vi "VisualizeNHRDC0.vi"() -> ()   [LabVIEW 2018, in "Visualization.lvlib" / "VisualizeAcPwr.lvclass"]
uses:
  VisualizeAcPwr.lvclass
  <vilib>/event_ctls.llb/usereventprio.ctl
  VisualizeBase/VisualizeBase_class/Requests/clUserEventType.ctl
  <vilib>/Utility/error.llb/Error Cluster From Error Code.vi
  <vilib>/ErrorRing/Error Ring.xnode
  VisualizeBase/VisualizeBase_class/VisualizeBase.lvclass
  <userlib>/NIST/NISTErrorLib/NISTErrorLib.lvlib
  AcPwr/AcPwrModule/AcPwrModule.lvlib
panel:
  out "Incorrect DataType?":bool
  in  "PluginName":string="AcPwr.NHRDC0"
  in  "PlotYAxis":u32[](array[numeric])=[0, 1, 0] max=1
  out "NHRDC":waveform(dbl)[](graph)
  out "ErrorArray":errorcluster[](array[cluster])
  in  "QueuName":string="NHRDCVQ"
  in  "btnStop":bool
  in  "btnReset":bool
  in  "btnClear":bool
  # "0=Left Axis and 1=Right Axis"
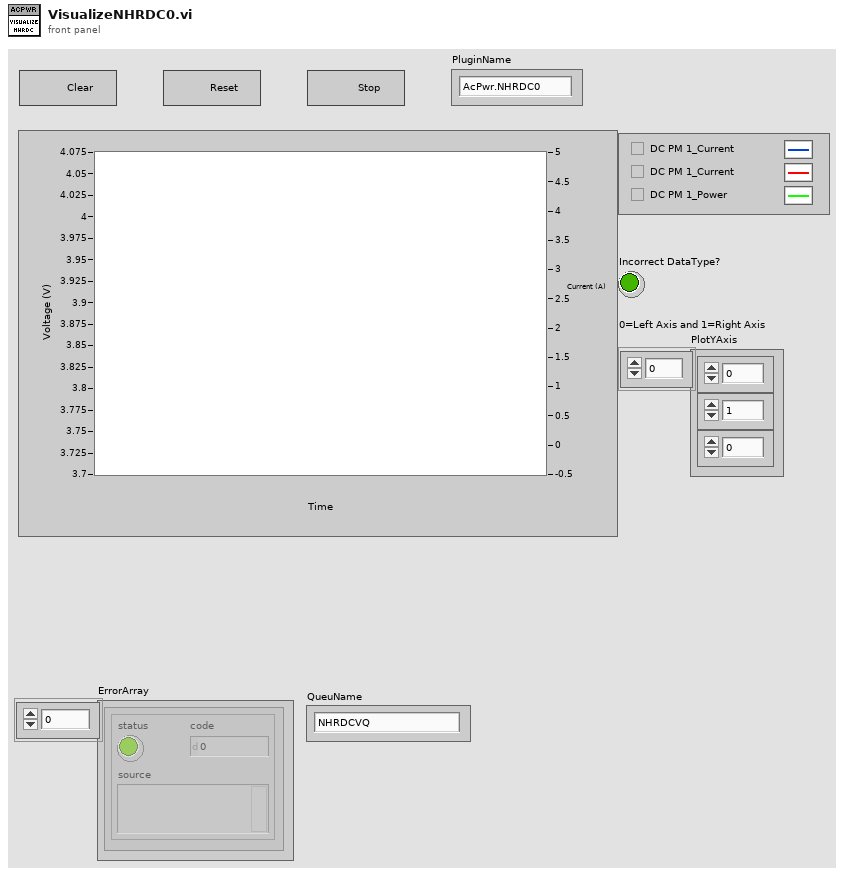
[diagram p1: front panel]
types:
  T1 = typedef "Visualization.lvlib/VisualizeBase.lvclass/clRequestEvents.ctl" = cluster{"StopRequest":refnum<user-event>, "ResetRequest":refnum<user-event>}
  T2 = typedef "AcPwrModule.lvlib/clBroadcastEvents.ctl" = cluster{"DidInit":refnum<user-event>, "StatusUpdate":refnum<user-event>, "ErrorReport":refnum<user-event>, "DidStop":refnum<user-event>, "PathToINI":refnum<user-event>, "Measurements":refnum<user-event>, "LoadConfigFile":refnum<user-event>, "GetSettings":refnum<user-event>, "SetSettings":refnum<user-event>, "GetType&ID":refnum<user-event>, "GotSettings":refnum<user-event>}
  T3 = typedef "Visualization.lvlib/VisualizeBase.lvclass/clUserEventType.ctl" = cluster{"BusIndex":i8, "Data":variant}
  T4 = typedef "usereventprio.ctl" = enum32{"high priority", "normal priority"}
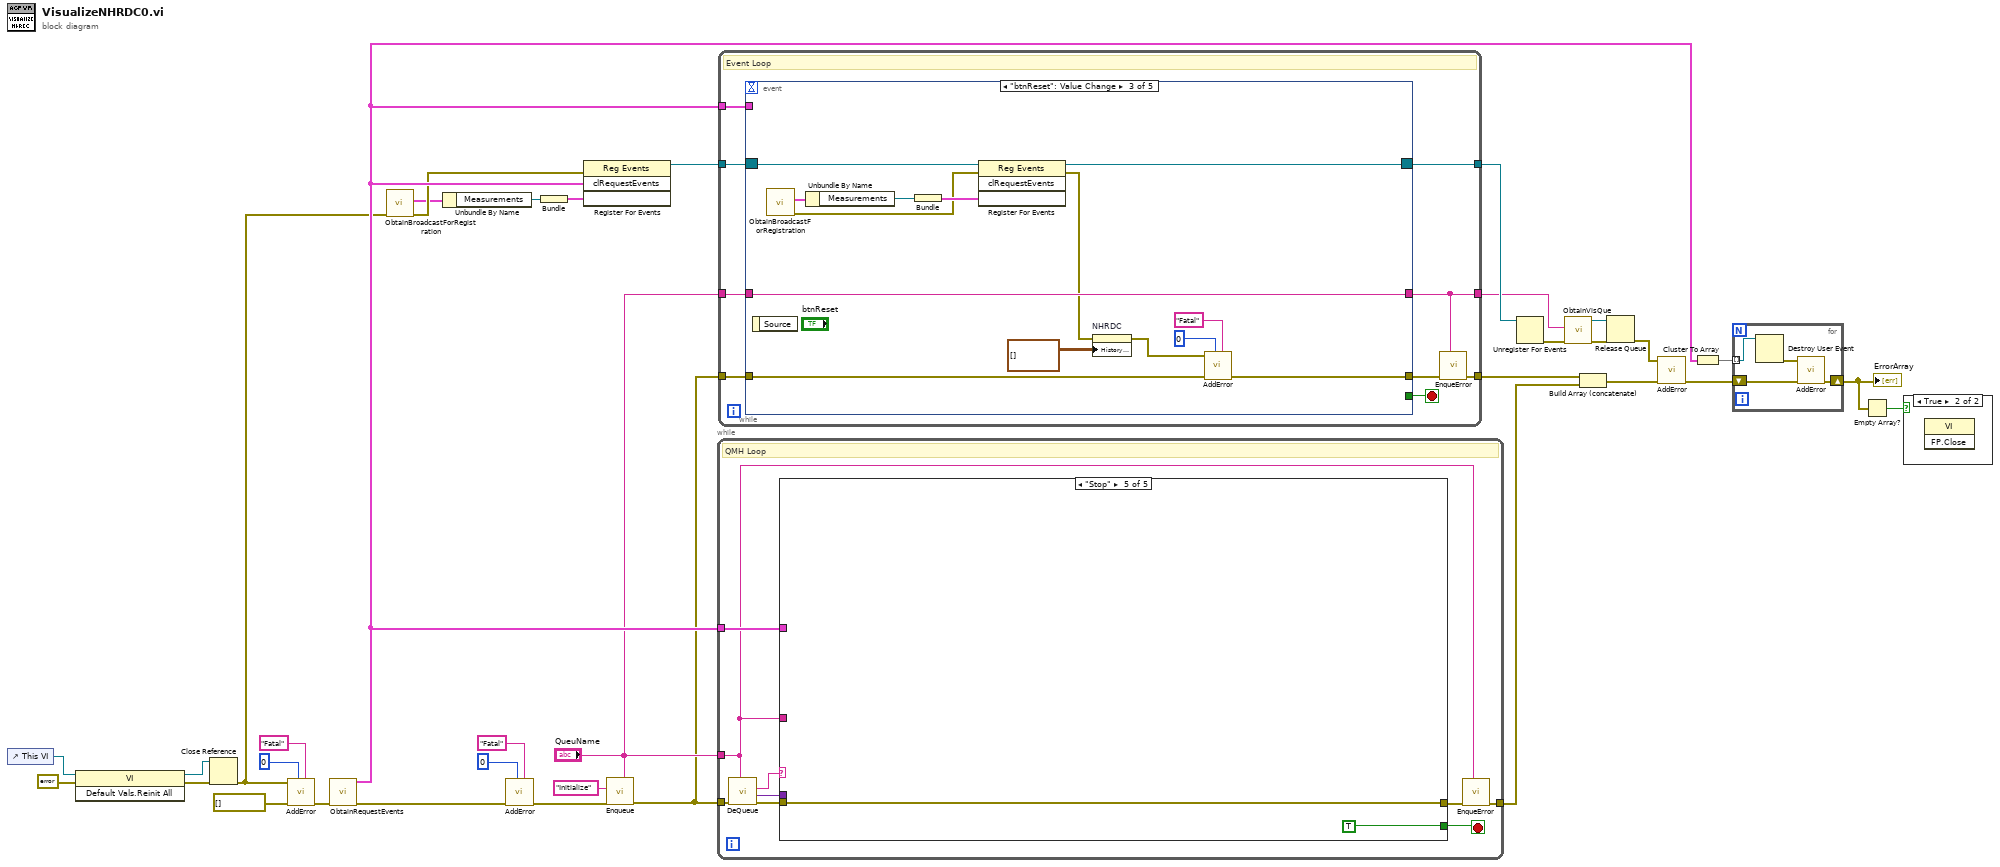
[diagram p0: block diagram]
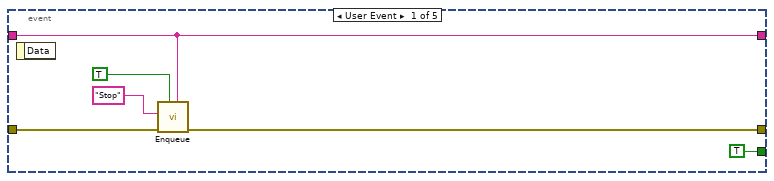
[diagram p2: hidden frame]
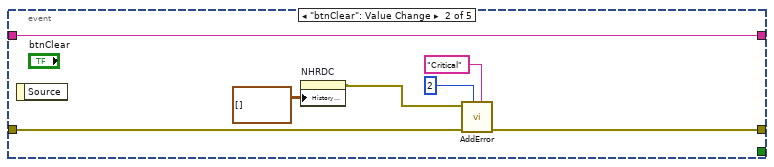
[diagram p3: hidden frame]
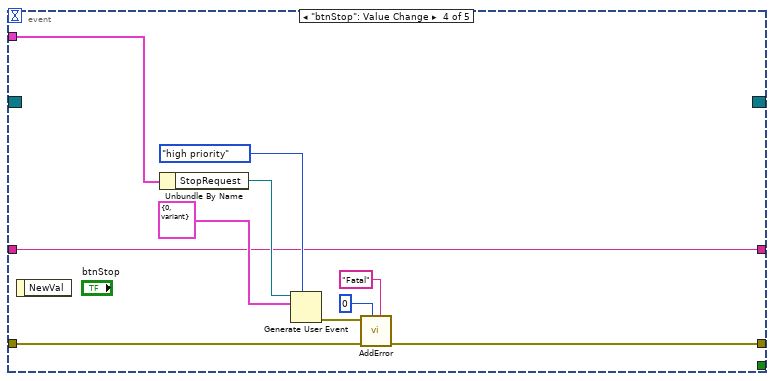
[diagram p4: hidden frame]
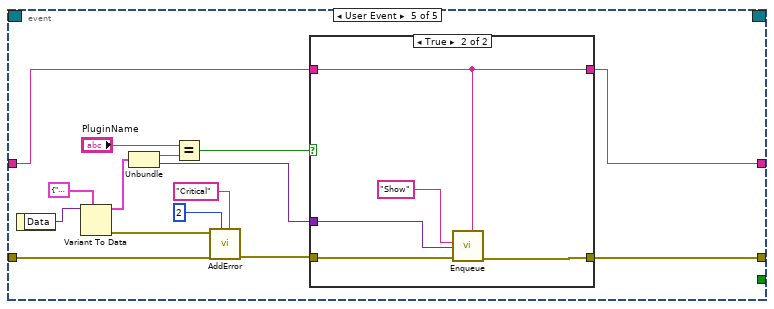
[diagram p5: hidden frame]
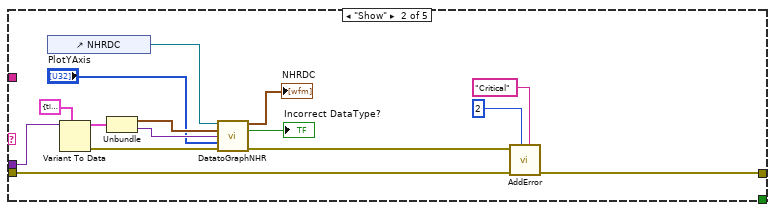
[diagram p8: hidden frame]
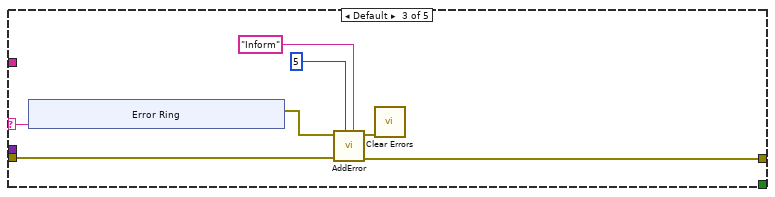
[diagram p9: hidden frame]
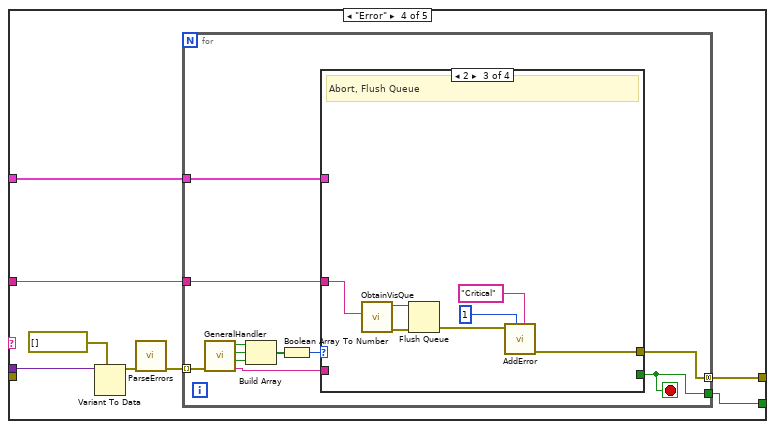
[diagram p10: hidden frame]
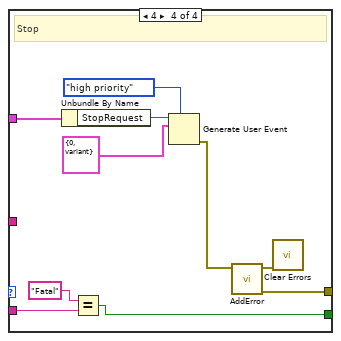
[diagram p13: hidden frame]
diagram:
  n1 = control-ref of="This VI"() -> (w18:refnum<vi>)
  n2 = invoke class="VI" method="Default Vals.Reinit All"(reference=w18, error in=errorcluster {"status"=FALSE, "code"=0, "source"=""} ("error in (no error)")) -> (reference out=w15:refnum<vi>, error out=w16:errorcluster)  [unwired: 1 in, 1 out]
  n3 = Close Reference(reference=w15, error in (no error)=w16) -> (error out=w13:errorcluster)
  n4 = call <userlib>:"AddError.vi"("Severity"="Fatal" ("String"), "Priority"=u8 0, "ErrorArray"=errorcluster[] [], "error in (no error)"=w13) -> ("ErrorArray"=w33:errorcluster[])  [unwired: 6 in, 1 out]
  n5 = call "ObtainRequestEvents.vi"("Error"=w33) -> ("Error"=w3:errorcluster[], "clRequestEvents"=w22:T1)  [unwired: 9 in]
  n6 = call "ObtainBroadcastForRegistration.vi"("error in (no error)"=w13) -> ("error out"=w12:errorcluster, "clBroadcastEvents"=w11:T2)  [unwired: 9 in]
  n7 = Unbundle By Name(w11) -> ("Measurements"=w20:refnum<user-event>)
  n8 = call <userlib>:"AddError.vi"("Severity"="Fatal" ("String"), "Priority"=u8 0, "ErrorArray"=w3) -> ("ErrorArray"=w2:errorcluster[])  [unwired: 7 in, 1 out]
  n9 = Bundle("Measurements"=w20) -> (w19:cluster{"Measurements":refnum<user-event>})  [unwired: 1 in]
  n10 = register-events(error in=w12, w22, w19) -> (reference out=w34:refnum<event-registration>)  [unwired: 1 in, 1 out]
  n11 = call "Enqueue.vi"("QueName"="QueuName", "Error"=w2, "Message"="Initialize") -> ("Error"=w1:errorcluster[])  [unwired: 8 in]
  n12 = while {
    tunnel: w1 -> [w44]
    tunnel: [w38] -> w29
    tunnel: "QueuName" -> [w36]
    tunnel: w22 -> [w37]
    stop <- w39 stop-if-true
    # "QMH Loop"
    n13 = call "DeQueue.vi"("QueName"=w36, "Error"=w44) -> ("Error"=w41:errorcluster[], "Data"=w42:variant, "Message"=w43:string)  [unwired: 7 in]
    n14 = case shown="\"Stop\"" w43 {
      selector: w43 -> [_ _ w67 _ _]
      tunnel: w42 -> [_ w53 _ w82 _]
      tunnel: w41 -> [w45 w56 w65 _ w111]
      tunnel: [w45 w60 w64 w78 w111] -> w40
      tunnel: [_ _ _ w77 TRUE] -> w39
      tunnel: w37 -> [_ _ _ w76 _]
      tunnel: w36 -> [_ _ _ w75 _]
      frame "Initialize" {
      }
      frame "Show" {
        n15 = control-ref of="NHRDC"() -> (w52:refnum<vi>)
        n16 = Variant To Data(type=cluster{timestamp, "Data":variant} {timestamp(0 s since 1904-01-01), "Data"=variant}, Variant=w53) -> (data=w55:cluster{timestamp, "Data":variant}, error out=w51:errorcluster)  [unwired: 1 in]
        n17 = Unbundle(w55) -> (w50:timestamp, "Data"=w49:variant)
        n18 = call "DatatoGraphNHR.vi"("NHRDC 2"=w52, "t0"=w50, "Data"=w49, "PlotYAxis"="PlotYAxis", "error in (no error)"=w51) -> ("WaveformArray"=→"NHRDC":waveform(dbl)[], "Incorrect DataType?"=→"Incorrect DataType?":bool, "error out"=w57:errorcluster)  [unwired: 8 in]
        n19 = call <userlib>:"AddError.vi"("Severity"="Critical" ("String"), "Priority"=u8 2, "ErrorArray"=w56, "error in (no error)"=w57) -> ("ErrorArray"=w60:errorcluster[])  [unwired: 6 in, 1 out]
      }
      frame Default {
        n20 = xnode "Error Ring"("parameter 0"=w67) -> ("error out"=w66:errorcluster)
        n21 = call <userlib>:"AddError.vi"("Severity"="Inform" ("String"), "Priority"=u8 5, "ErrorArray"=w65, "error in (no error)"=w66) -> ("ErrorArray"=w64:errorcluster[], "error out"=w63:errorcluster)  [unwired: 6 in]
        n22 = call <vilib>:"Clear Errors.vi"("error in (no error)"=w63) -> ()  [unwired: 5 in, 2 out]
      }
      frame "Error" {
        n23 = Variant To Data(type=errorcluster[] [], Variant=w82) -> (data=w80:errorcluster[])  [unwired: 1 in, 1 out]
        n24 = call <userlib>:"ParseErrors.vi"("ErrorArray"=w80) -> ("ErrorArray"=w79:errorcluster[])  [unwired: 8 in, 2 out]
        n25 = for {
          tunnel: w79 -> [w93] mode=indexing
          tunnel: [w87] -> w78 mode=concatenating
          tunnel: [w85] -> w77
          tunnel: w76 -> [w84]
          tunnel: w75 -> [w83]
          stop <- w85 stop-if-true
          n26 = call <userlib>:"GeneralHandler.vi"("error in (no error)"=w93) -> ("Severity"=w86:string, "Stop"=w90:bool, "Abort"=w91:bool, "Continue"=w92:bool)  [unwired: 7 in]
          n27 = Build Array(w92, w91, w90) -> (w89:bool[])
          n28 = Boolean Array To Number(Boolean array=w89) -> (number=w88:u32)
          n29 = case shown="2" w88 {
            tunnel: [_ _ w98 w109] -> w87
            tunnel: w86 -> [_ _ _ w104]
            tunnel: [_ _ _ w102] -> w85
            tunnel: w84 -> [_ _ _ w101]
            tunnel: w83 -> [_ _ w94 _]
            frame 0, Default {
              # "No Dialog"
            }
            frame 1 {
              # "Continue"
            }
            frame 2 {
              # "Abort, Flush Queue"
              n30 = call "ObtainVisQue.vi"("QueName"=w94) -> ("error out"=w100:errorcluster, "queue out"=w99:refnum<queue>)  [unwired: 9 in]
              n31 = Flush Queue(queue=w99, error in (no error)=w100) -> (error out=w97:errorcluster)  [unwired: 2 out]
              n32 = call <userlib>:"AddError.vi"("Severity"="Critical" ("String"), "Priority"=u8 1, "error in (no error)"=w97) -> ("ErrorArray"=w98:errorcluster[])  [unwired: 7 in, 1 out]
            }
            frame 4 {
              # "Stop"
              n33 = Unbundle By Name(w101) -> ("StopRequest"=w110:refnum<user-event>)
              n34 = Equal?(x="Fatal", y=w104) -> (x = y?=w102:bool)
              n35 = Generate User Event(priority (normal)=usereventprio."high priority", user event=w110, event data cluster=T3 {"BusIndex"=0, "Data"=variant} ("event data")) -> (error out=w108:errorcluster)  [unwired: 1 in, 1 out]
              n36 = call <userlib>:"AddError.vi"("error in (no error)"=w108) -> ("ErrorArray"=w109:errorcluster[], "error out"=w105:errorcluster)  [unwired: 9 in]
              n37 = call <vilib>:"Clear Errors.vi"("error in (no error)"=w105) -> ()  [unwired: 5 in, 2 out]
            }
          }
        }
      }
      frame "Stop" {
      }
    }
    n38 = call "EnqueError.vi"("QueName"=w36, "Error"=w40) -> ("Error"=w38:errorcluster[])  [unwired: 9 in]
  }
  n39 = while {
    tunnel: w34 -> [w121]
    tunnel: [w118] -> w30
    tunnel: [w117] -> w32
    tunnel: w22 -> [w116]
    tunnel: w1 -> [w115]
    tunnel: "QueuName" -> [w114]
    tunnel: [w113] -> w9
    stop <- w120 stop-if-true
    # "Event Loop"
    n40 = event shown="[2] \"btnReset\": Value Change" {
      selector: w121 -> [_ _ w148 _ _]
      dyn-events: [_ _ w147 _ _] -> w117
      timeout: _ -> [_ _ _ _ _]
      tunnel: [TRUE _ _ _ _] -> w120
      tunnel: [w126 w131 w141 w156 w173] -> w119
      tunnel: w116 -> [_ _ _ w151 _]
      tunnel: w115 -> [w123 w130 w140 w149 w160]
      tunnel: w114 -> [w122 w134 w142 w150 w166]
      tunnel: [w122 w134 w142 w150 w165] -> w113
      event User Event {
        n41 = event-data() -> ()  [unwired: 1 in, 1 out]
        n42 = call "Enqueue.vi"("QueName"=w122, "Priority? (F)"=TRUE, "Error"=w123, "Message"="Stop") -> ("Error"=w126:errorcluster[])  [unwired: 7 in]
      }
      event "btnClear": Value Change {
        n43 = event-data() -> ()  [unwired: 1 in, 1 out]
        n44 = property on="NHRDC" class="WFChart (strict)"("History Data"=waveform(dbl)[][] []) -> (error out=w128:errorcluster)  [unwired: 2 in, 1 out]
        n45 = call <userlib>:"AddError.vi"("Severity"="Critical" ("String"), "Priority"=u8 2, "ErrorArray"=w130, "error in (no error)"=w128) -> ("ErrorArray"=w131:errorcluster[])  [unwired: 6 in, 1 out]
      }
      event "btnReset": Value Change {
        n46 = event-data() -> ()  [unwired: 1 in, 1 out]
        n47 = call "ObtainBroadcastForRegistration.vi"() -> ("error out"=w143:errorcluster, "clBroadcastEvents"=w144:T2)  [unwired: 10 in]
        n48 = Unbundle By Name(w144) -> ("Measurements"=w146:refnum<user-event>)
        n49 = Bundle("Measurements"=w146) -> (w145:cluster{"Measurements":refnum<user-event>})  [unwired: 1 in]
        n50 = register-events(reference=w148, error in=w143, w145) -> (reference out=w147:refnum<event-registration>, error out=w136:errorcluster)  [unwired: 1 in]
        n51 = property on="NHRDC" class="WFChart (strict)"(error in=w136, "History Data"=waveform(dbl)[][] []) -> (error out=w135:errorcluster)  [unwired: 1 in, 1 out]
        n52 = call <userlib>:"AddError.vi"("Severity"="Fatal" ("String"), "Priority"=u8 0, "ErrorArray"=w140, "error in (no error)"=w135) -> ("ErrorArray"=w141:errorcluster[])  [unwired: 6 in, 1 out]
      }
      event "btnStop": Value Change {
        n53 = event-data() -> ()  [unwired: 1 in, 1 out]
        n54 = Unbundle By Name(w151) -> ("StopRequest"=w157:refnum<user-event>)
        n55 = Generate User Event(priority (normal)=usereventprio."high priority", user event=w157, event data cluster=T3 {"BusIndex"=0, "Data"=variant} ("event data")) -> (error out=w158:errorcluster)  [unwired: 1 in, 1 out]
        n56 = call <userlib>:"AddError.vi"("Severity"="Fatal" ("String"), "Priority"=u8 0, "ErrorArray"=w149, "error in (no error)"=w158) -> ("ErrorArray"=w156:errorcluster[])  [unwired: 6 in, 1 out]
      }
      event User Event {
        n57 = event-data() -> ("Data"=w168:variant)  [unwired: 1 in]
        n58 = Variant To Data(type=cluster{string, "Data":variant} {"", "Data"=variant}, Variant=w168) -> (data=w171:cluster{string, "Data":variant}, error out=w159:errorcluster)  [unwired: 1 in]
        n59 = Unbundle(w171) -> (w170:string, "Data"=w164:variant)
        n60 = Equal?(x="PluginName", y=w170) -> (x = y?=w167:bool)
        n61 = call <userlib>:"AddError.vi"("Severity"="Critical" ("String"), "Priority"=u8 2, "ErrorArray"=w160, "error in (no error)"=w159) -> ("ErrorArray"=w161:errorcluster[])  [unwired: 6 in, 1 out]
        n62 = case shown="True" w167 {
          tunnel: w164 -> [_ w180]
          tunnel: [w175 w178] -> w173
          tunnel: w161 -> [w175 w177]
          tunnel: w166 -> [w174 w176]
          tunnel: [w174 w176] -> w165
          frame False {
          }
          frame True {
            n63 = call "Enqueue.vi"("QueName"=w176, "Error"=w177, "Data"=w180, "Message"="Show") -> ("Error"=w178:errorcluster[])  [unwired: 7 in]
          }
        }
      }
    }
    n64 = call "EnqueError.vi"("QueName"=w113, "Error"=w119) -> ("Error"=w118:errorcluster[])  [unwired: 9 in]
  }
  n65 = Unregister For Events(event registration refnum=w32) -> (error out=w28:errorcluster)  [unwired: 1 in]
  n66 = call "ObtainVisQue.vi"("error in (no error)"=w28, "QueName"=w9) -> ("error out"=w26:errorcluster, "queue out"=w25:refnum<queue>)  [unwired: 8 in]
  n67 = Build Array (concatenate)(w30, w29) -> (w27:errorcluster[])
  n68 = Release Queue(queue=w25, error in (no error)=w26) -> (error out=w24:errorcluster)  [unwired: 1 in, 2 out]
  n69 = call <userlib>:"AddError.vi"("ErrorArray"=w27, "error in (no error)"=w24) -> ("ErrorArray"=w23:errorcluster[])  [unwired: 8 in, 1 out]
  n70 = Cluster To Array(cluster=w22) -> (array=w31:refnum<user-event>[])
  n71 = for {
    tunnel: w31 -> [w184] mode=indexing
    shift-right: [w183] -> w14
    shift-left: w23 -> [w182]
    n72 = Destroy User Event(user event=w184) -> (error out=w181:errorcluster)  [unwired: 1 in]
    n73 = call <userlib>:"AddError.vi"("ErrorArray"=w182, "error in (no error)"=w181) -> ("ErrorArray"=w183:errorcluster[])  [unwired: 8 in, 1 out]
  }
  "ErrorArray" <- w14
  n74 = Empty Array?(array=w14) -> (empty?=w21:bool)
  n75 = case shown="True" w21 {
    frame False {
    }
    frame True {
      n76 = invoke class="VI" method="FP.Close"() -> ()  [unwired: 3 in, 3 out]
    }
  }
